vi "items.vi"(8 "error in (no error)":errorcluster, 11 "reference in":refnum<class "Project Panels.lvclass">=refnum) -> (0 "error out":errorcluster={"status"=TRUE, "code"=1556, "source"="In Place Element Structure in Project Panels.lvclass:items.vi"}, 2 "saved?":bool, 3 "reference out":refnum<class "Project Panels.lvclass">)   [LabVIEW 2015, in "Project Panels.lvclass"]
uses:
  Project Panels.lvclass
  SYS/Items Controller_llb/storageSheets.ctl
  stateItem.ctl
  <vilib>/Utility/miscctls.llb/LVRowAndColumnUnsignedTypeDef.ctl
  <vilib>/Utility/miscctls.llb/LVRowAndColumnTypeDef.ctl
  SYS/Items Controller_llb/Items Controller.lvclass
  SYS/File Controller_llb/File Controller.lvclass
panel:
  out "title":string="Cosmed Asia Pacific - Storage"
  in  "tables":enum32{"Check IN", "Check OUT", "Storage"}(tab)
  in  "checkIN":string[][](table)
  in  "checkOUT":string[][](table)
  in  "Storage":string[][](table)
  in  "uploadFile":bool
  in  "Add Check OUT":bool
  in  "Add Check IN":bool
  out "Number of Items:":i32
  out "index":i32
  in  "back":bool
  in  "next":bool
  out "storageSheets":T1
  in  "Search Item":bool
  in  "Save":bool
  out "Item Selected (S/N or P/N):":string
  out "statuBar":string="Stoped for an Error"
  in  "Stop Button":bool
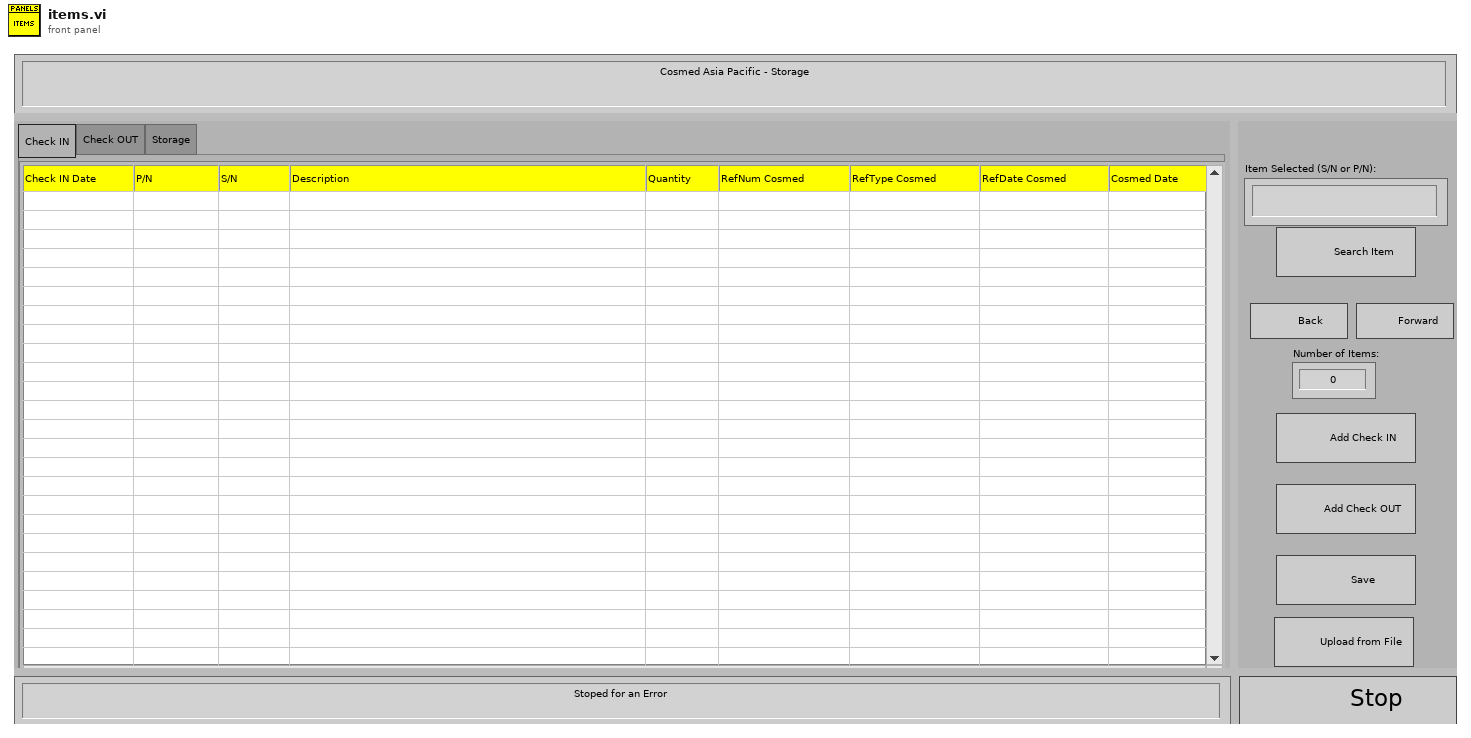
[diagram p1: front panel]
types:
  T1 = typedef "Items Controller.lvclass/storageSheets.ctl" = enum16{"check-in", "check-out", "storage"}
  T2 = typedef "Project Panels.lvclass/stateItem.ctl" = enum16{"initiate", "waitEvent", "save", "search", "UploadFile", "nextItems", "stop"}
  T3 = typedef "LVRowAndColumnUnsignedTypeDef.ctl" = cluster{"Row":u32, "Column":u32}
  T4 = enum8{"Enabled", "Disabled", "Disabled and Grayed Out"}
  T5 = cluster{"checkIN":string[][], "checkOUT":string[][], "storage":string[][]}
  T6 = typedef "LVRowAndColumnTypeDef.ctl" = cluster{"Row":i32, "Column":i32}
  T7 = typedef "Project Panels.lvclass/ObjectAttributesRef.ctl" = refnum<data-value>
  T8 = typedef "Project Panels.lvclass/ObjectAttributes.ctl" = cluster{"MyAttribute":dbl, "device_controller_ref":refnum<class "Devices Controller.lvclass">, "file_controller_ref":refnum<class "File Controller.lvclass">, "item_controller_ref":refnum<class "Items Controller.lvclass">, "item_tables":cluster{"checkIN":string[][], "checkOUT":string[][], "storage":string[][]}, "quickbook_table":cluster{"notes":string[][]}, "notification_controller_ref":refnum<class "Notification Controller.lvclass">, "partstracking_controller_ref":refnum<class "PartsTracking Controller.lvclass">, "product_tables":cluster{"k4b2":string[][], "fitmate":string[][], "RMR":string[][], "CPET":string[][], "BP":string[][], "PP":string[][], "k5":string[][], "bb-pft":string[][]}, "rowsColour":u32[], "low_resolution?":bool}
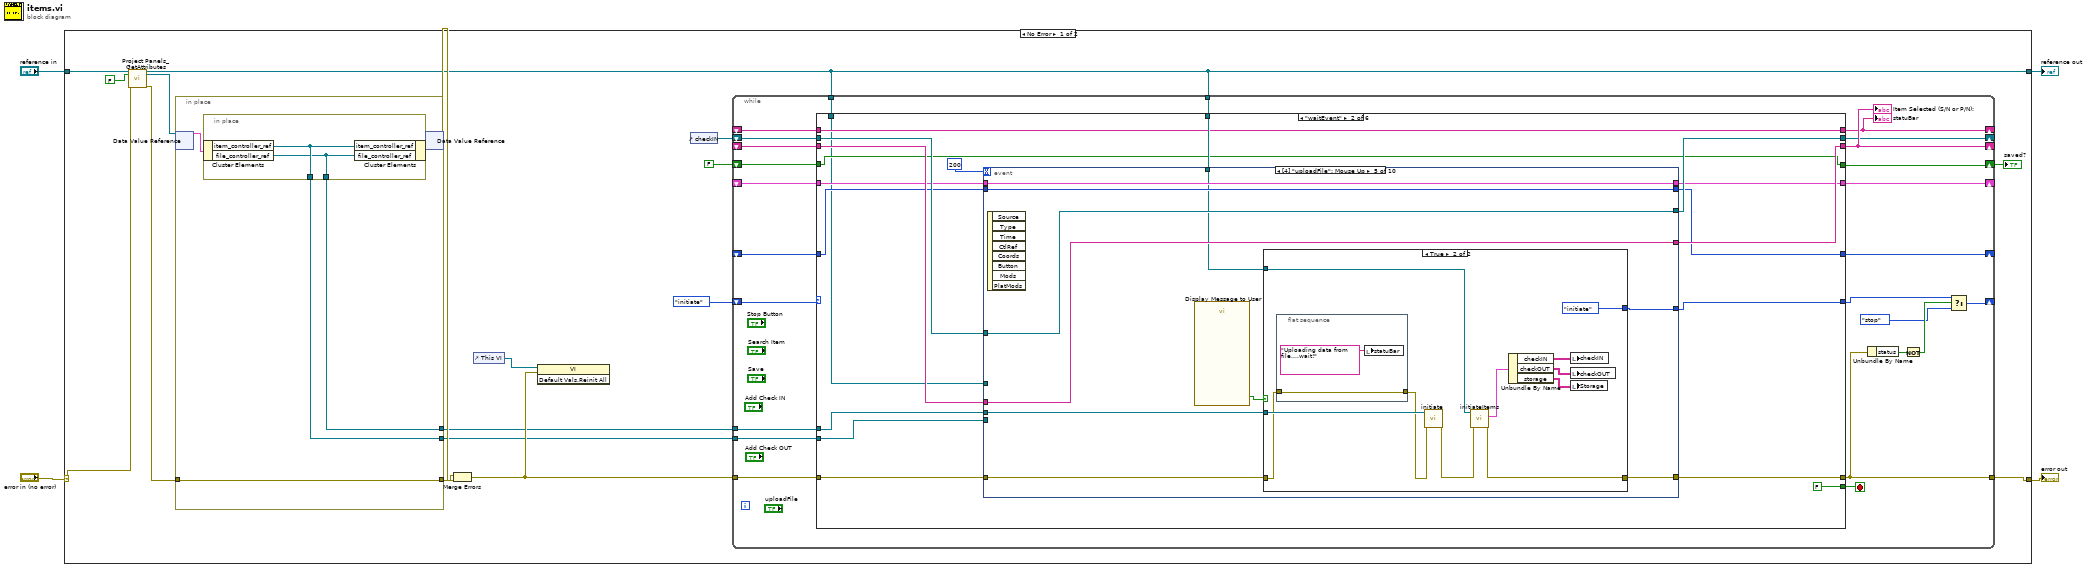
[diagram p0: block diagram]
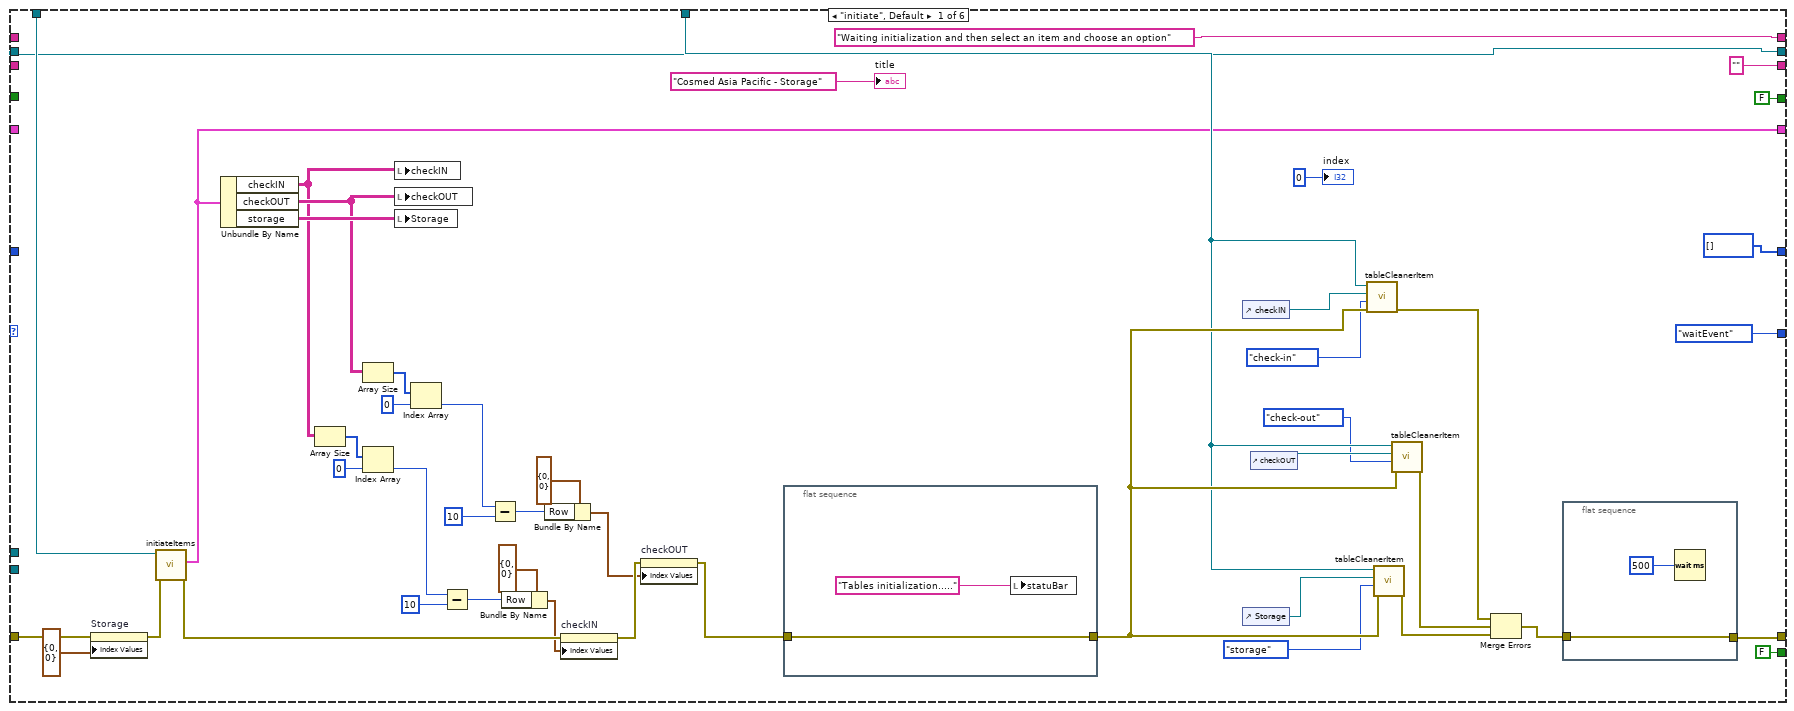
[diagram p2: hidden frame]
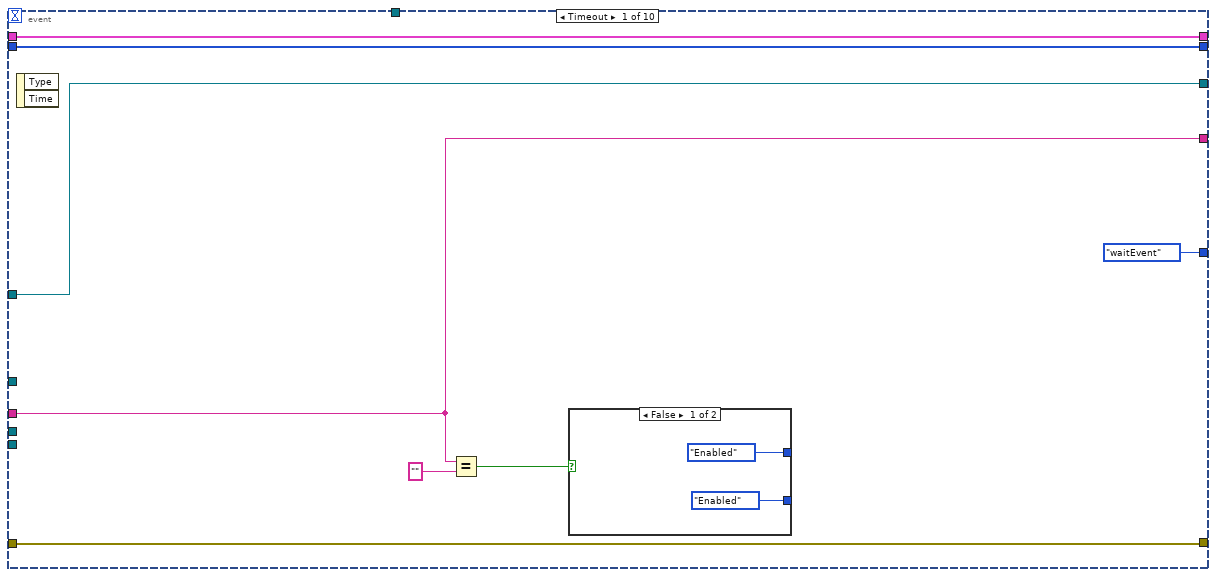
[diagram p3: hidden frame]
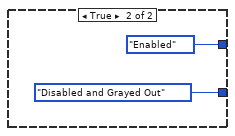
[diagram p4: hidden frame]
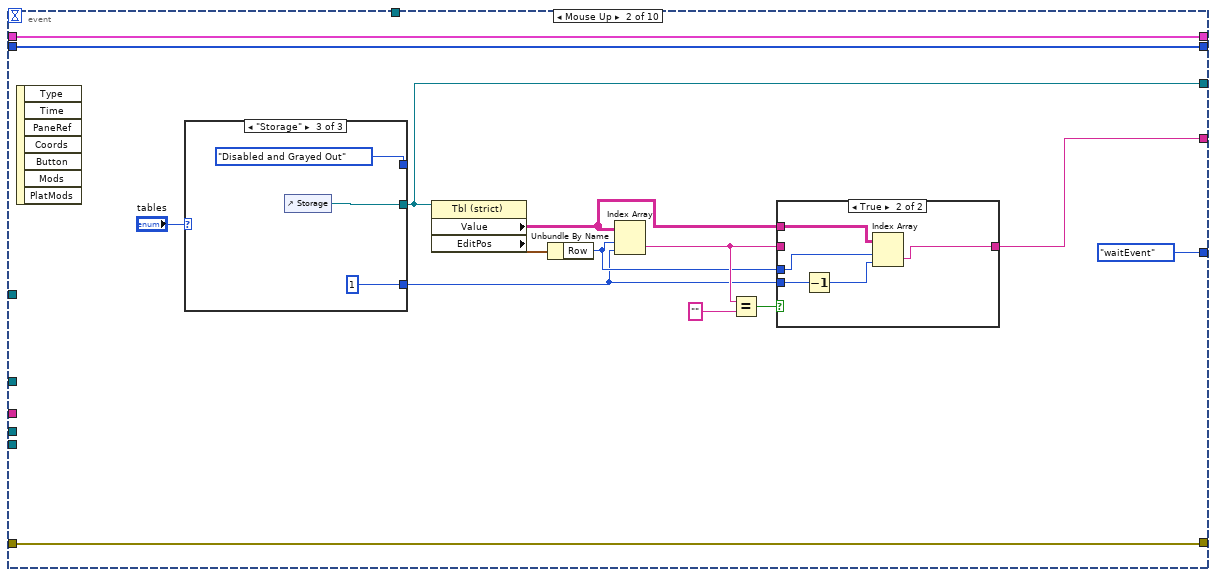
[diagram p5: hidden frame]
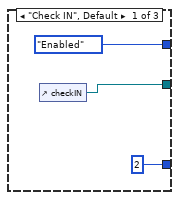
[diagram p7: hidden frame]
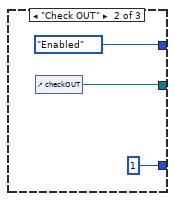
[diagram p8: hidden frame]
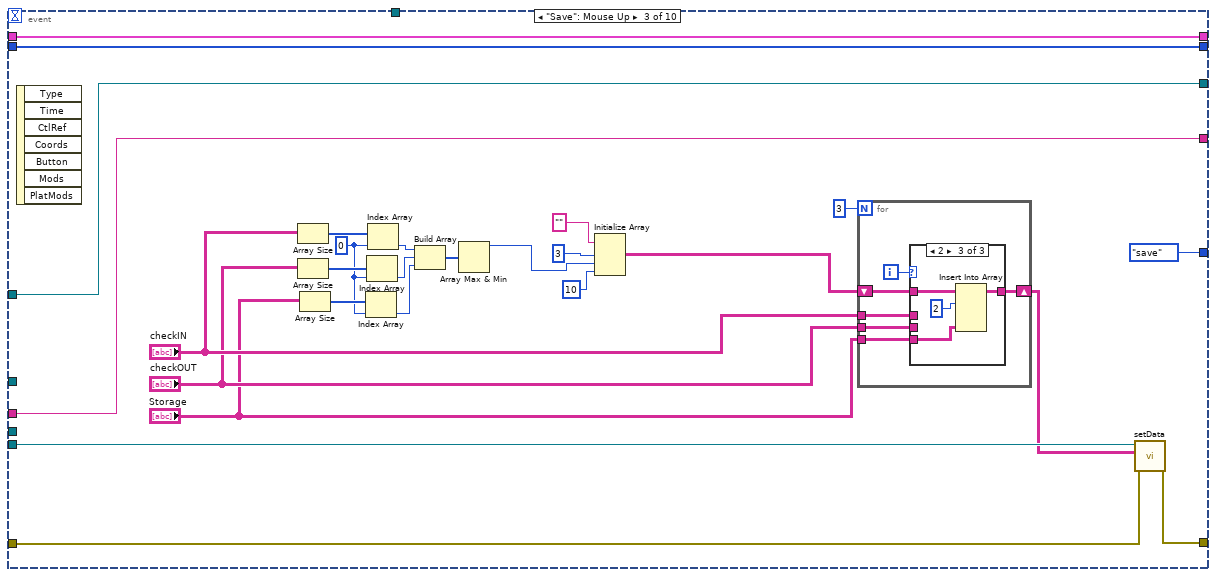
[diagram p9: hidden frame]
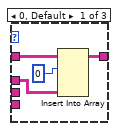
[diagram p10: hidden frame]
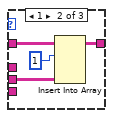
[diagram p11: hidden frame]
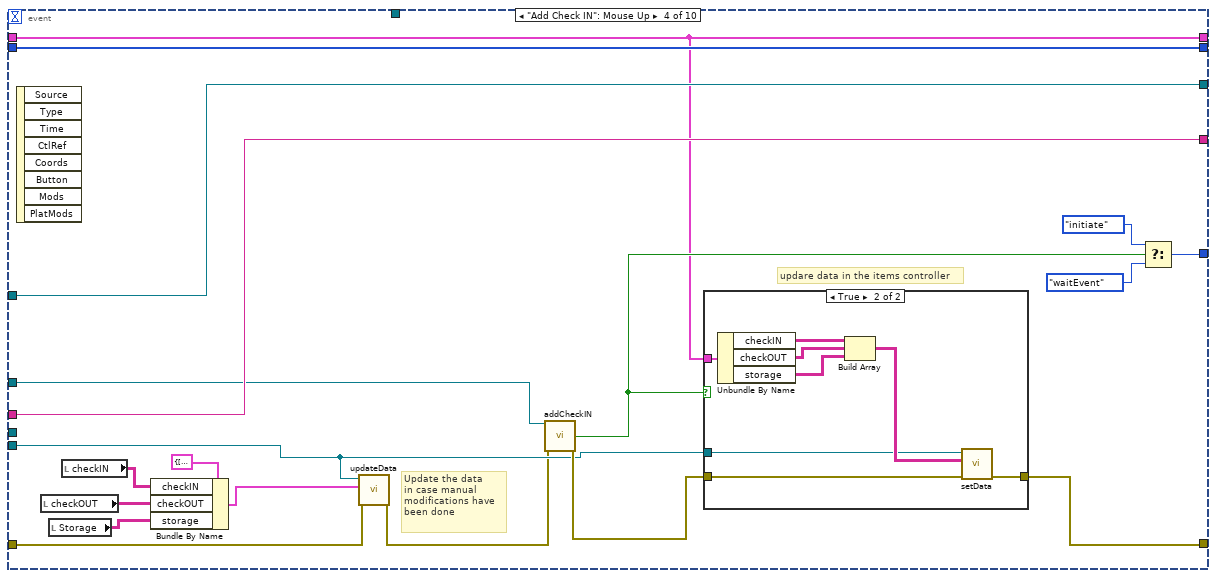
[diagram p12: hidden frame]
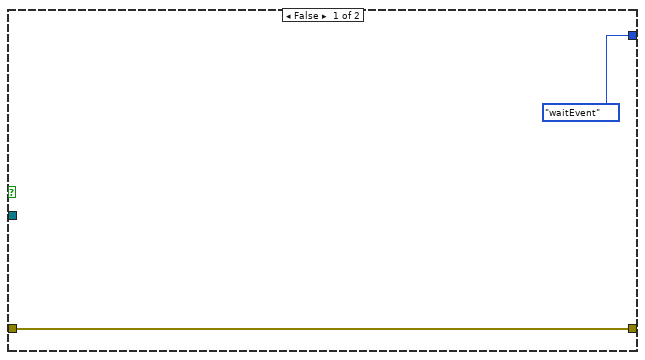
[diagram p14: hidden frame]
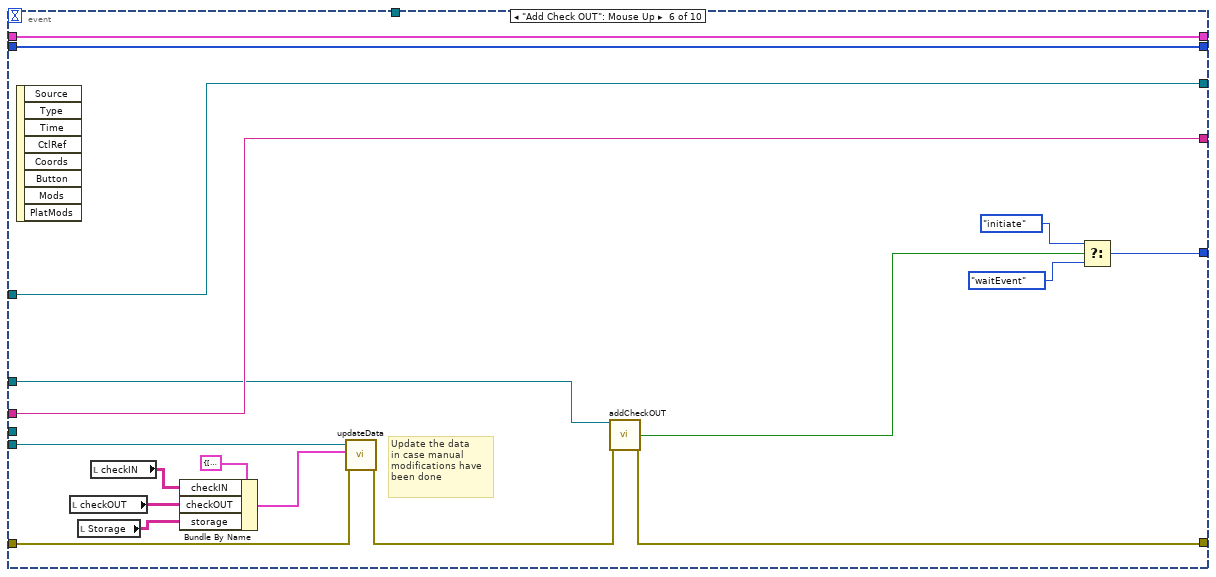
[diagram p15: hidden frame]
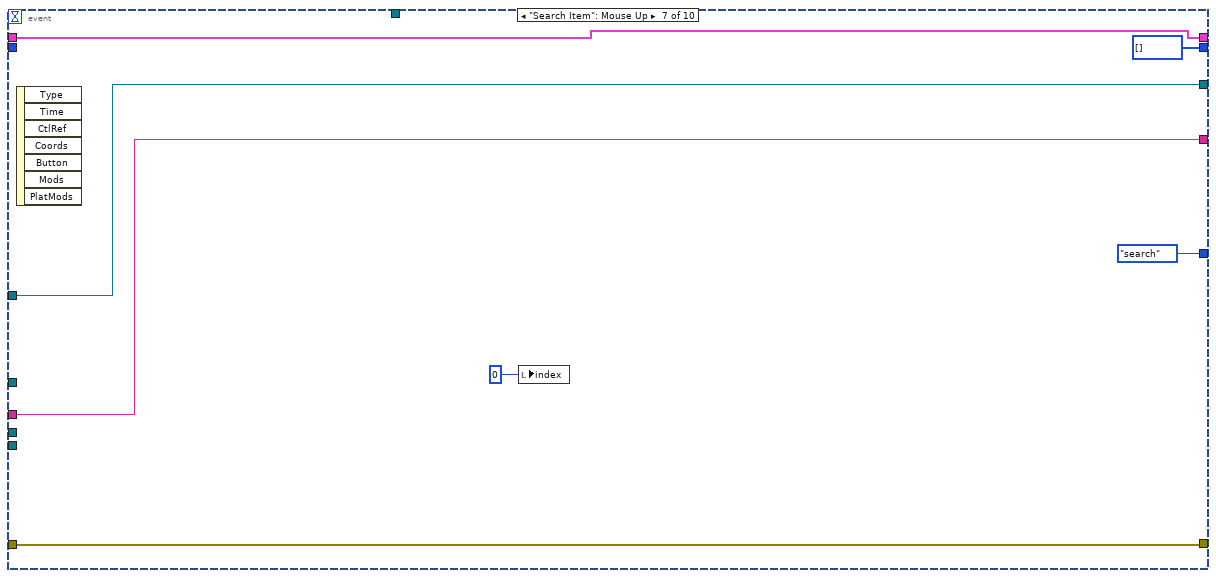
[diagram p16: hidden frame]
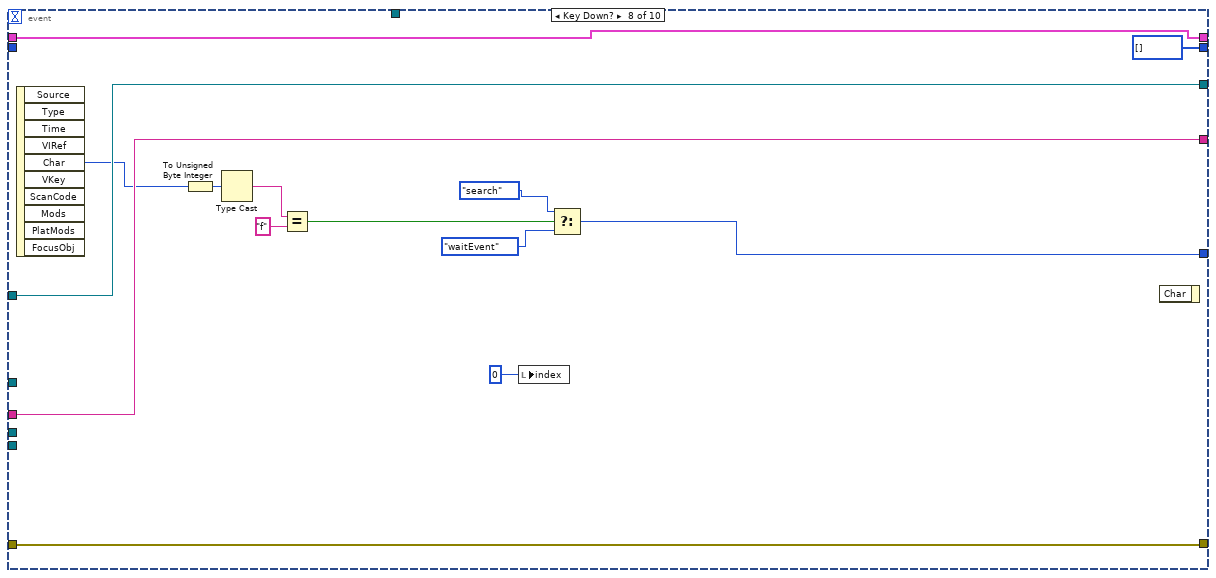
[diagram p17: hidden frame]
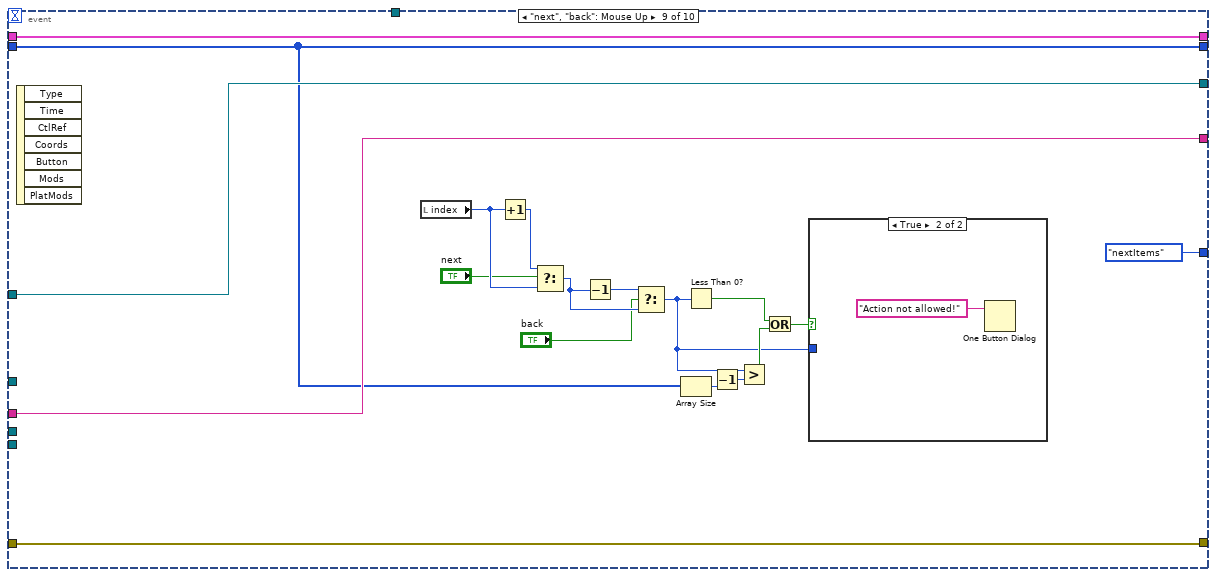
[diagram p18: hidden frame]
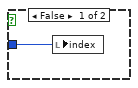
[diagram p19: hidden frame]
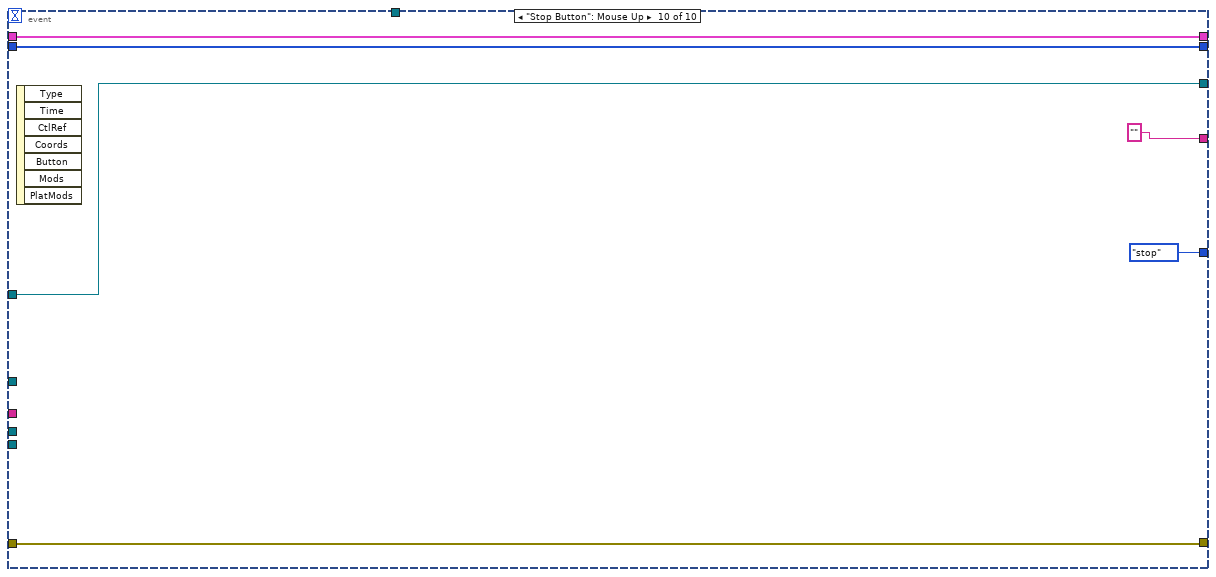
[diagram p20: hidden frame]
diagram:
  n1 = case shown="No Error" "error in (no error)" {
    selector: "error in (no error)" -> [w17 w412]
    tunnel: [w14 w412] -> w3
    tunnel: [w12 w411] -> w1
    tunnel: "reference in" -> [w19 w411]
    frame No Error {
      n2 = call "Project Panels_GetAttributes.vi"("reference in"=w19, "return data? (T)"=FALSE, "error in (no error)"=w17) -> ("reference out"=w12:refnum<class "Project Panels.lvclass">, "attributes ref"=w15:T7, "error out"=w16:errorcluster)  [unwired: 13 in, 1 out]
      n3 = in-place {
        in-place-border: w16 -> [w406]
        in-place-border: [w406] -> w20
        in-place-border: [w405] -> w8
        in-place-border: [w404] -> w5
        n4 = in-place-dvr #1(w15) -> (w407:T8)  [unwired: 1 out]
        n5 = in-place {
          in-place-border: [w410] -> w405
          in-place-border: [w409] -> w404
          n6 = in-place-cluster #2(w407) -> ("item_controller_ref"=w410:refnum<class "Items Controller.lvclass">, "file_controller_ref"=w409:refnum<class "File Controller.lvclass">)
          n7 = in-place-cluster #2("item_controller_ref"=w410, "file_controller_ref"=w409) -> (w408:T8)
        }
        n8 = in-place-dvr #1(w408) -> (w21:errorcluster)  [unwired: 1 out]
      }
      n9 = Merge Errors(w20, w21) -> (w9:errorcluster)
      n10 = control-ref of="This VI"() -> (w10:refnum<vi>)
      n11 = invoke class="VI" method="Default Vals.Reinit All"(reference=w10, error in=w9) -> ()  [unwired: 1 in, 3 out]
      n12 = control-ref of="checkIN"() -> (w11:refnum<vi>)
      n13 = while {
        tunnel: w12 -> [w46]
        tunnel: w9 -> [w45]
        tunnel: [w43] -> w14
        shift-right: [w40] -> _
        shift-left: stateItem."initiate" ("state") -> [w44]
        shift-right: [w37] -> _
        shift-left: _ -> [w36]
        shift-right: [w35] -> _
        shift-left: w11 -> [w34]
        tunnel: w12 -> [w33]
        tunnel: w8 -> [w31]
        shift-right: [w29] -> w6
        shift-left: FALSE -> [w30]
        shift-right: [w28] -> _
        shift-left: _ -> [w27]
        shift-right: [w26] -> _
        shift-left: _ -> [w25]
        shift-right: [w24] -> _
        shift-left: _ -> [w23]
        tunnel: w5 -> [w22]
        stop <- w38 stop-if-true
        n14 = case shown="\"waitEvent\"" w44 {
          tunnel: w46 -> [w81 w106 _ _ _ _]
          tunnel: w45 -> [w74 w115 w330 w348 w380 w394]
          tunnel: [w84 w109 w330 w359 w380 w389] -> w43
          tunnel: [stateItem."waitEvent" ("state") w108 w325 w354 stateItem."waitEvent" ("state") stateItem."waitEvent" ("state")] -> w41
          tunnel: [FALSE FALSE w323 FALSE FALSE FALSE] -> w38
          tunnel: ["Waiting initialization and then select an item and choose an option" ("title") w104 w332 "Search Item option selected..." ("title") "Click on the arrows to select other items" ("title") w388] -> w28
          tunnel: ["" w111 w335 w360 w377 w396] -> w37
          tunnel: w36 -> [_ w113 w335 w360 w377 w396]
          tunnel: [w78 w110 w331 w361 w371 w397] -> w35
          tunnel: w34 -> [w78 w112 w331 w361 w371 w397]
          tunnel: w33 -> [w80 w99 _ w350 _ _]
          tunnel: w31 -> [_ w107 _ _ _ w395]
          tunnel: w30 -> [_ w105 w322 w358 w378 _]
          tunnel: [FALSE w105 w322 w358 w378 TRUE] -> w29
          tunnel: w27 -> [_ w104 _ _ _ _]
          tunnel: [i32[] [] ("indexElements") w102 w321 w352 w372 w391] -> w26
          tunnel: w25 -> [_ w103 w321 _ w372 w391]
          tunnel: [w47 w100 w320 w349 w364 w387] -> w24
          tunnel: w23 -> [_ w101 w320 w349 w364 w387]
          tunnel: w22 -> [_ w98 _ _ _ _]
          frame "initiate", Default {
            n15 = property on="Storage" class="Tbl (strict)"(error in=w74, "Index Values"=T3 {"Row"=0, "Column"=0}) -> (error out=w73:errorcluster)  [unwired: 1 in, 1 out]
            n16 = call "initiateItems.vi"("error in (no error)"=w73, "reference in"=w80) -> ("error out"=w65:errorcluster, "table"=w47:T5)  [unwired: 7 in, 1 out]
            n17 = Unbundle By Name(w47) -> ("checkIN"=w48:string[][], "checkOUT"=w67:string[][], "storage"=w72:string[][])
            n18 = Array Size(array=w48) -> (size(s)=w54:i32[])
            n19 = Array Size(array=w67) -> (size(s)=w61:i32[])
            n20 = Index Array(array=w54, index=0) -> (element=w51:i32)
            n21 = local write "checkIN"(w48) -> ()
            n22 = local write "checkOUT"(w67) -> ()
            n23 = local write "Storage"(w72) -> ()
            n24 = Index Array(array=w61, index=0) -> (element=w58:i32)
            n25 = Subtract(x=w51, y=10) -> (x-y=w52:i32)
            n26 = Subtract(x=w58, y=10) -> (x-y=w59:i32)
            n27 = Bundle By Name(cluster=T3 {"Row"=0, "Column"=0} ("Index Values"), "Row"=w52) -> (w49:T3)
            n28 = Bundle By Name(cluster=T3 {"Row"=0, "Column"=0} ("Index Values"), "Row"=w59) -> (w56:T3)
            n29 = property on="checkIN" class="Tbl (strict)"(error in=w65, "Index Values"=w49) -> (error out=w64:errorcluster)  [unwired: 1 in, 1 out]
            n30 = property on="checkOUT" class="Tbl (strict)"(error in=w64, "Index Values"=w56) -> (error out=w66:errorcluster)  [unwired: 1 in, 1 out]
            n31 = flat-sequence {
              tunnel: w66 -> [w95]
              tunnel: [w95] -> w83
              frame #0 {
                n32 = local write "statuBar"("Tables initialization....." ("title")) -> ()
              }
            }
            n33 = control-ref of="checkIN"() -> (w91:refnum<vi>)
            n34 = control-ref of="Storage"() -> (w93:refnum<vi>)
            n35 = control-ref of="checkOUT"() -> (w92:refnum<vi>)
            n36 = call "tableCleanerItem.vi"("error in (no error)"=w83, "storageSheets"=storageSheets."check-in", "Table in"=w91, "reference in"=w81) -> ("error out"=w90:errorcluster)  [unwired: 6 in, 1 out]
            n37 = call "tableCleanerItem.vi"("error in (no error)"=w83, "storageSheets"=storageSheets."storage", "Table in"=w93, "reference in"=w81) -> ("error out"=w88:errorcluster)  [unwired: 6 in, 1 out]
            n38 = call "tableCleanerItem.vi"("error in (no error)"=w83, "storageSheets"=storageSheets."check-out", "Table in"=w92, "reference in"=w81) -> ("error out"=w89:errorcluster)  [unwired: 6 in, 1 out]
            n39 = Merge Errors(w90, w89, w88) -> (w79:errorcluster)
            n40 = flat-sequence {
              tunnel: w79 -> [w97]
              tunnel: [w97] -> w84
              frame #0 {
                n41 = Wait (ms)(milliseconds to wait=u32 500) -> ()  [unwired: 1 out]
              }
            }
            "title" <- "Cosmed Asia Pacific - Storage" ("title")
            "index" <- 0 ("index")
          }
          frame "waitEvent" {
            n42 = event shown="[4] \"uploadFile\": Mouse Up" {
              selector: _ -> [_ _ _ _ _ _ _ _ _ _]
              dyn-events: _ -> [_ _ _ _ _ _ _ _ _ _]
              timeout: 200 -> [_ _ _ _ _ _ _ _ _ _]
              tunnel: w115 -> [w124 w142 w179 w208 w235 w263 w276 w291 w311 w319]
              tunnel: [w124 w142 w178 w211 w234 w268 w276 w291 w311 w319] -> w109
              tunnel: w113 -> [w120 _ w182 w220 w236 w272 w278 w292 w304 _]
              tunnel: w112 -> [w121 _ w183 w219 w237 w271 w279 w293 w305 w317]
              tunnel: [w120 w135 w182 w220 w236 w272 w278 w292 w304 ""] -> w111
              tunnel: [w121 w139 w183 w219 w237 w271 w279 w293 w305 w317] -> w110
              tunnel: [stateItem."waitEvent" ("state") stateItem."waitEvent" ("state") stateItem."save" ("state") w215 w232 w266 stateItem."search" ("state") w281 stateItem."nextItems" ("state") stateItem."stop" ("state")] -> w108
              tunnel: w107 -> [_ _ w177 w210 _ w261 _ _ _ _]
              tunnel: w106 -> [_ _ _ _ w230 _ _ _ _ _]
              tunnel: w103 -> [w118 w130 w175 w218 w238 w270 _ _ w303 w315]
              tunnel: [w118 w130 w175 w218 w238 w270 i32[] [] ("indexElements") i32[] [] ("indexElements") w303 w315] -> w102
              tunnel: w101 -> [w117 w129 w174 w209 w239 w260 w273 w288 w294 w314]
              tunnel: [w117 w129 w174 w209 w239 w260 w273 w288 w294 w314] -> w100
              tunnel: w99 -> [_ _ _ w217 _ w269 _ _ _ _]
              tunnel: w98 -> [_ _ _ _ w231 _ _ _ _ _]
              event Timeout {
                n43 = event-data() -> ()  [unwired: 1 in, 2 out]
                n44 = Equal?(x=w120, y="") -> (x = y?=w123:bool)
                n45 = case shown="False" w123 {
                  tunnel: [T4."Enabled" ("Disabled") T4."Disabled and Grayed Out" ("Disabled")] -> _
                  tunnel: [T4."Enabled" ("Disabled") T4."Enabled" ("Disabled")] -> _
                  frame False {
                  }
                  frame True {
                  }
                }
              }
              event Mouse Up {
                n46 = event-data() -> ()  [unwired: 1 in, 7 out]
                n47 = case shown="\"Storage\"" "tables" {
                  tunnel: [w151 w154 w157] -> w139
                  tunnel: [T4."Enabled" ("Disabled") T4."Enabled" ("Disabled") T4."Disabled and Grayed Out" ("Disabled")] -> _
                  tunnel: [2 ("disabled index (col)") 1 ("disabled index (col)") 1 ("disabled index (col)")] -> w132
                  frame "Check IN", Default {
                    n48 = control-ref of="checkIN"() -> (w151:refnum<vi>)
                  }
                  frame "Check OUT" {
                    n49 = control-ref of="checkOUT"() -> (w154:refnum<vi>)
                  }
                  frame "Storage" {
                    n50 = control-ref of="Storage"() -> (w157:refnum<vi>)
                  }
                }
                n51 = property on="Property Node" class="Tbl (strict)"(reference=w139) -> ("Value"=w134:string[][], "EditPos"=w141:T6)  [unwired: 1 in, 2 out]
                n52 = Unbundle By Name(w141) -> ("Row"=w133:i32)
                n53 = Index Array(array=w134, index (row)=w133, index (col)=w132) -> (element=w136:string)
                n54 = Equal?(x=w136, y="") -> (x = y?=w137:bool)
                n55 = case shown="True" w137 {
                  tunnel: w136 -> [w143 _]
                  tunnel: [w143 w144] -> w135
                  tunnel: w134 -> [_ w148]
                  tunnel: w133 -> [_ w147]
                  tunnel: w132 -> [_ w146]
                  frame False {
                  }
                  frame True {
                    n56 = Decrement(x=w146) -> (x-1=w145:i32)
                    n57 = Index Array(array=w148, index (row)=w147, index (col)=w145) -> (element=w144:string)
                  }
                }
              }
              event "Save": Mouse Up {
                w167 = 0 ("index")
                n58 = event-data() -> ()  [unwired: 1 in, 7 out]
                n59 = Array Size(array="checkIN") -> (size(s)=w170:i32[])
                n60 = Array Size(array="checkOUT") -> (size(s)=w169:i32[])
                n61 = Array Size(array="Storage") -> (size(s)=w168:i32[])
                n62 = Index Array(array=w168, index=w167) -> (element=w164:i32)
                n63 = Index Array(array=w169, index=w167) -> (element=w165:i32)
                n64 = Index Array(array=w170, index=w167) -> (element=w166:i32)
                n65 = Build Array(w166, w165, w164) -> (w163:i32[])
                n66 = Array Max & Min(array=w163) -> (max value=w160:i32)  [unwired: 3 out]
                n67 = Initialize Array("", 3 ("dimension size"), w160, 10 ("dimension size")) -> (w158:string[][][])
                n68 = for {
                  N: 3 -> [_]
                  shift-right: [w186] -> w176
                  shift-left: w158 -> [w188]
                  tunnel: "checkIN" -> [w187]
                  tunnel: "checkOUT" -> [w185]
                  tunnel: "Storage" -> [w184]
                  i -> [w189]
                  n69 = case shown="2" w189 {
                    tunnel: w188 -> [w193 w197 w201]
                    tunnel: w187 -> [w190 _ _]
                    tunnel: [w192 w196 w200] -> w186
                    tunnel: w185 -> [_ w194 _]
                    tunnel: w184 -> [_ _ w198]
                    frame 0, Default {
                      n70 = Insert Into Array(array=w193, index (dim 0)=0 ("index (page)"), new element=w190) -> (w192:string[][][])  [unwired: 2 in]
                    }
                    frame 1 {
                      n71 = Insert Into Array(array=w197, index (dim 0)=1 ("disabled index (page)"), new element=w194) -> (w196:string[][][])  [unwired: 2 in]
                    }
                    frame 2 {
                      n72 = Insert Into Array(array=w201, index (dim 0)=2 ("disabled index (page)"), new element=w198) -> (w200:string[][][])  [unwired: 2 in]
                    }
                  }
                }
                n73 = call "setData.vi"("error in (no error)"=w179, "data"=w176, "reference in"=w177) -> ("error out"=w178:errorcluster)  [unwired: 7 in, 1 out]
              }
              event "Add Check IN": Mouse Up {
                # "Update the data\nin case manual\nmodifications have\nbeen done"
                # "updare data in the items controller"
                n74 = event-data() -> ()  [unwired: 1 in, 8 out]
                n75 = local read "checkOUT"() -> (w204:string[][])
                n76 = local read "Storage"() -> (w203:string[][])
                n77 = local read "checkIN"() -> (w205:string[][])
                n78 = Bundle By Name(cluster=T5 {"checkIN"=[], "checkOUT"=[], "storage"=[]} ("table"), "checkIN"=w205, "checkOUT"=w204, "storage"=w203) -> (w202:T5)
                n79 = call "updateData.vi"("error in (no error)"=w208, "table"=w202, "reference in"=w210) -> ("error out"=w207:errorcluster)  [unwired: 7 in, 1 out]
                n80 = call "addCheckIN.vi"("reference in"=w217, "error in (no error)"=w207) -> ("saved?"=w213:bool, "error out"=w212:errorcluster)  [unwired: 11 in, 1 out]
                n81 = case shown="True" w213 {
                  tunnel: w209 -> [_ w225]
                  tunnel: w212 -> [w221 w224]
                  tunnel: [w221 w223] -> w211
                  tunnel: w210 -> [_ w222]
                  frame False {
                  }
                  frame True {
                    n82 = Unbundle By Name(w225) -> ("checkIN"=w229:string[][], "checkOUT"=w228:string[][], "storage"=w227:string[][])
                    n83 = Build Array(w229, w228, w227) -> (w226:string[][][])
                    n84 = call "setData.vi"("error in (no error)"=w224, "data"=w226, "reference in"=w222) -> ("error out"=w223:errorcluster)  [unwired: 7 in, 1 out]
                  }
                }
                n85 = Select(t=stateItem."initiate" ("state"), s=w213, f=stateItem."waitEvent") -> (s? t:f=w215:T2)
              }
              event "uploadFile": Mouse Up {
                n86 = event-data() -> ()  [unwired: 1 in, 8 out]
                n87 = call "Display Message to User"() -> ("Yes"=w233:bool)  [unwired: 10 in, 1 out]
                n88 = case shown="True" w233 {
                  tunnel: w235 -> [w241 w243]
                  tunnel: [w241 w247] -> w234
                  tunnel: [stateItem."waitEvent" ("state") stateItem."initiate" ("state")] -> w232
                  tunnel: w231 -> [_ w251]
                  tunnel: w230 -> [_ w249]
                  frame False {
                  }
                  frame True {
                    n89 = flat-sequence {
                      tunnel: w243 -> [w254]
                      tunnel: [w254] -> w242
                      frame #0 {
                        n90 = local write "statuBar"("Uploading data from file....wait!" ("statuBar")) -> ()
                      }
                    }
                    n91 = call "initiate.vi"("reference in"=w251, "error in (no error)"=w242) -> ("error out"=w248:errorcluster)  [unwired: 16 in, 1 out]
                    n92 = call "initiateItems.vi"("error in (no error)"=w248, "reference in"=w249) -> ("error out"=w247:errorcluster, "table"=w250:T5)  [unwired: 7 in, 1 out]
                    n93 = Unbundle By Name(w250) -> ("checkIN"=w246:string[][], "checkOUT"=w245:string[][], "storage"=w244:string[][])
                    n94 = local write "checkIN"(w246) -> ()
                    n95 = local write "checkOUT"(w245) -> ()
                    n96 = local write "Storage"(w244) -> ()
                  }
                }
              }
              event "Add Check OUT": Mouse Up {
                # "Update the data\nin case manual\nmodifications have\nbeen done"
                n97 = event-data() -> ()  [unwired: 1 in, 8 out]
                n98 = local read "checkOUT"() -> (w257:string[][])
                n99 = local read "Storage"() -> (w256:string[][])
                n100 = local read "checkIN"() -> (w258:string[][])
                n101 = Bundle By Name(cluster=T5 {"checkIN"=[], "checkOUT"=[], "storage"=[]} ("table"), "checkIN"=w258, "checkOUT"=w257, "storage"=w256) -> (w255:T5)
                n102 = call "updateData.vi"("error in (no error)"=w263, "table"=w255, "reference in"=w261) -> ("error out"=w262:errorcluster)  [unwired: 7 in, 1 out]
                n103 = call "addCheckOUT.vi"("reference in"=w269, "error in (no error)"=w262) -> ("saved?"=w265:bool, "error out"=w268:errorcluster)  [unwired: 11 in, 1 out]
                n104 = Select(t=stateItem."initiate" ("state"), s=w265, f=stateItem."waitEvent") -> (s? t:f=w266:T2)
              }
              event "Search Item": Mouse Up {
                n105 = event-data() -> ()  [unwired: 1 in, 7 out]
                n106 = local write "index"(0 ("index")) -> ()
              }
              event Key Down? {
                n107 = event-data() -> ("Char"=w286:i16)  [unwired: 1 in, 9 out]
                n108 = To Unsigned Byte Integer(number=w286) -> (unsigned 8bit integer=w287:u8)
                n109 = Type Cast(x=w287) -> (*(type *) &x=w285:string)  [unwired: 1 in]
                n110 = Equal?(x=w285, y="f") -> (x = y?=w280:bool)
                n111 = local write "index"(0 ("index")) -> ()
                n112 = Select(t=stateItem."search" ("state"), s=w280, f=stateItem."waitEvent" ("state")) -> (s? t:f=w281:T2)
                n113 = event-data() -> ()  [unwired: 2 in, 1 out]
              }
              event "next", "back": Mouse Up {
                n114 = event-data() -> ()  [unwired: 1 in, 7 out]
                n115 = local read "index"() -> (w309:i32)
                n116 = Increment(x=w309) -> (x+1=w310:i32)
                n117 = Select(t=w310, s="next", f=w309) -> (s? t:f=w307:i32)
                n118 = Decrement(x=w307) -> (x-1=w308:i32)
                n119 = Select(t=w308, s="back", f=w307) -> (s? t:f=w298:i32)
                n120 = Array Size(array=w303) -> (size(s)=w302:i32)
                n121 = Less Than 0?(x=w298) -> (x < 0?=w300:bool)
                n122 = Decrement(x=w302) -> (x-1=w295:i32)
                n123 = Greater?(x=w298, y=w295) -> (0:w301:bool)
                n124 = Or(x=w300, y=w301) -> (x .or. y?=w299:bool)
                n125 = case shown="True" w299 {
                  tunnel: w298 -> [w312 _]
                  frame False {
                    n126 = local write "index"(w312) -> ()
                  }
                  frame True {
                    n127 = One Button Dialog(message="Action not allowed!") -> ()  [unwired: 1 in, 1 out]
                  }
                }
              }
              event "Stop Button": Mouse Up {
                n128 = event-data() -> ()  [unwired: 1 in, 7 out]
              }
            }
          }
          frame "stop" {
            n129 = Unbundle By Name(w330) -> ("status"=w329:bool)
            n130 = Not(x=w329) -> (.not. x?=w328:bool)
            n131 = case shown="False" w329 {
              tunnel: w330 -> [_ w345]
              tunnel: [w337 FALSE ("Save")] -> w324
              tunnel: w322 -> [w336 _]
              frame False {
                n132 = case shown="False" w336 {
                  tunnel: [w340 FALSE ("Save")] -> w337
                  frame False {
                    n133 = Two Button Dialog(message="The panel will be closed without saving the data. Do you want to save the data?", 1:"Not Save" ("F button name (\"Cancel\")"), 2:"Save" ("T button name (\"OK\")")) -> (T button?=w340:bool)
                  }
                  frame True {
                  }
                }
              }
              frame True {
                n134 = Unbundle By Name(w345) -> ("source"=w344:string)
                n135 = Concatenate Strings("An Error occur: " ("message"), w344) -> (w347:string)
                n136 = One Button Dialog(message=w347) -> ()  [unwired: 1 in, 1 out]
              }
            }
            n137 = Select(t="Stoped from User" ("title"), s=w328, f="Stoped for an Error" ("title")) -> (s? t:f=w332:string)
            n138 = Not(x=w324) -> (.not. x?=w323:bool)
            n139 = Select(t=stateItem."save", s=w324, f=stateItem."stop" ("state")) -> (s? t:f=w325:T2)
          }
          frame "search" {
            n140 = call "searchItem.vi"("reference in"=w350, "error in (no error)"=w348) -> ("Sheet out"=→"storageSheets":T1, "indexElements"=w352:i32[], "error out"=w359:errorcluster)  [unwired: 10 in, 1 out]
            n141 = Array Size(array=w352) -> (size(s)=w351:i32)
            "Number of Items:" <- w351
            n142 = Greater Than 0?(x=w351) -> (x > 0?=w353:bool)
            n143 = Select(t=stateItem."nextItems" ("state"), s=w353, f=stateItem."waitEvent" ("state")) -> (s? t:f=w354:T2)
          }
          frame "nextItems" {
            n144 = local read "storageSheets"() -> (w367:T1)
            n145 = local read "index"() -> (w374:i32)
            n146 = case shown="\"storage\"" w367 {
              tunnel: [w382 w384 w386] -> w366
              tunnel: [enum32{"Check IN", "Check OUT", "Storage"}."Check IN" ("tables") enum32{"Check IN", "Check OUT", "Storage"}."Check OUT" ("tables") enum32{"Check IN", "Check OUT", "Storage"}."Storage" ("tables")] -> w365
              frame "check-in", Default {
                n147 = control-ref of="checkIN"() -> (w382:refnum<vi>)
              }
              frame "check-out" {
                n148 = control-ref of="checkOUT"() -> (w384:refnum<vi>)
              }
              frame "storage" {
                n149 = control-ref of="Storage"() -> (w386:refnum<vi>)
              }
            }
            n150 = Index Array(array=w372, index=w374) -> (element=w373:i32)
            n151 = Bundle By Name(cluster=T6 {"Row"=0, "Column"=0} ("Active Cell:Active Cell"), "Row"=w373, "Column"=0) -> (w368:T6)
            n152 = local write "tables"(w365) -> ()
            n153 = property on="Property Node" class="Tbl (strict)"(reference=w366, "Index Values"=w368) -> ()  [unwired: 1 in, 2 out]
          }
          frame "save" {
            n154 = flat-sequence {
              tunnel: w394 -> [w403]
              tunnel: [w403] -> w393
              frame #0 {
                n155 = local write "statuBar"("Saving...wait" ("title")) -> ()
              }
            }
            n156 = call "saveData.vi"("error in (no error)"=w393, "reference in"=w395) -> ("error out"=w390:errorcluster)  [unwired: 8 in, 1 out]
            n157 = flat-sequence {
              tunnel: w390 -> [w401]
              tunnel: [w401] -> w389
              tunnel: ["select an item and choose an option" ("title")] -> w388
              frame #0 {
              }
            }
          }
        }
        "statuBar" <- w28
        "Item Selected (S/N or P/N):" <- w37
        n158 = Unbundle By Name(w43) -> ("status"=w42:bool)
        n159 = Not(x=w42) -> (.not. x?=w39:bool)
        n160 = Select(t=w41, s=w39, f=stateItem."stop" ("state")) -> (s? t:f=w40:T2)
      }
      "saved?" <- w6
    }
    frame Error {
    }
  }
  "error out" <- w3
  "reference out" <- w1
